vi "ActionVIOnCompile.vi"(8 "error in (no error)":errorcluster, 11 "Device Item Ref in":T1 format="%.0x") -> (0 "error out":errorcluster)   [LabVIEW 2019, in "NI-SWITCH System Explorer.lvlib"]
uses:
  NI-SWITCH System Explorer.lvlib
  <vilib>/NI VeriStand/Custom Device API/Custom Device Item Ref.ctl
  Shared/Compiled.Settings.ctl
  Shared/Communication Configuration.ctl
  Shared/Driver Configuration.ctl
  Shared/FIFO Indices.ctl
  Shared/Constants.vi
  <vilib>/NI VeriStand/Custom Device API/Set Item Property (Variant).vi
  <vilib>/NI VeriStand/Custom Device API/Custom Device API.lvlib
  Shared/NI-SWITCH Shared.lvlib
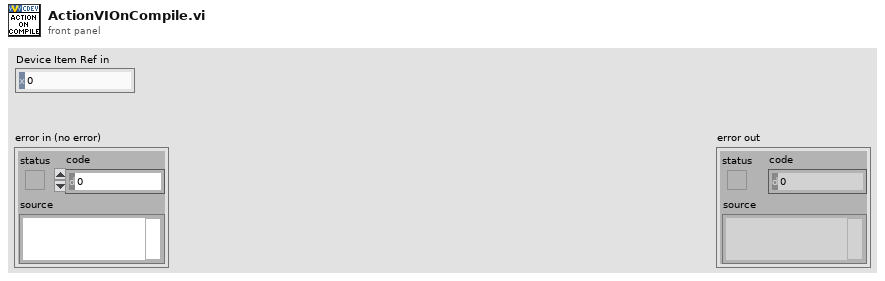
[diagram p1: front panel]
types:
  T1 = typedef "Custom Device API.lvlib/Custom Device Item Ref.ctl" = u64
  T2 = typedef "NI-SWITCH Shared.lvlib/Compiled.Settings.ctl" = cluster{"Custom Device Name":string, "Communication Configuration":T3, "Driver Configuration":T4, "FIFO Indices":T5}
  T3 = typedef "NI-SWITCH Shared.lvlib/Communication Configuration.ctl" = cluster{"Consumer Queue Name":string}
  T4 = typedef "NI-SWITCH Shared.lvlib/Driver Configuration.ctl" = cluster{"Topology":string, "Resource":string, "Source Channels":string[], "Configuration Channels":string[]}
  T5 = typedef "NI-SWITCH Shared.lvlib/FIFO Indices.ctl" = cluster{"Status Channel":i32, "Heartbeat Channel":i32}
  T6 = typedef "Custom Device API.lvlib/Custom Device Item Info.ctl" = cluster{"Name":string, "Is Channel":bool, "GUID":string, "Is Waveform":bool}
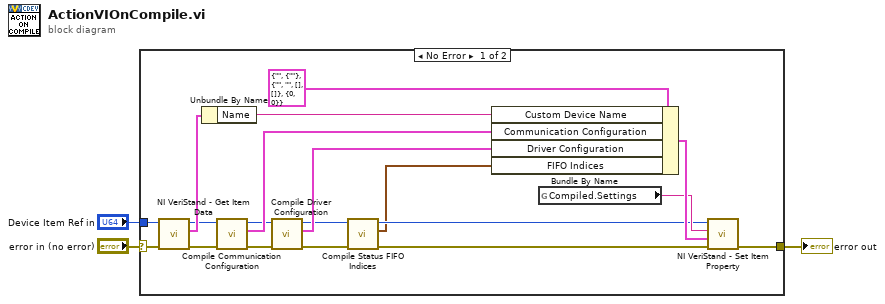
[diagram p0: block diagram]
diagram:
  n1 = case shown="No Error" "error in (no error)" {
    selector: "error in (no error)" -> [w21 w23]
    tunnel: [w22 w23] -> w2
    tunnel: "Device Item Ref in" -> [w20 _]
    frame No Error {
      n2 = call <vilib>:"NI VeriStand - Get Item Data.vi"("error in (no error)"=w21, "Item Ref in"=w20) -> ("error out"=w13:errorcluster, "Item Info"=w19:T6, "Item Ref out"=w14:T1)  [unwired: 6 in, 1 out]
      n3 = Unbundle By Name(w19) -> ("Name"=w18:string)
      n4 = call "Compile Communication Configuration.vi"("error in (no error)"=w13, "Device Ref in"=w14) -> ("error out"=w12:errorcluster, "Communication Configuration"=w11:T3, "Device Ref out"=w10:T1)  [unwired: 7 in]
      n5 = call "Compile Driver Configuration.vi"("error in (no error)"=w12, "Device Ref in"=w10) -> ("error out"=w8:errorcluster, "Driver Configuration"=w16:T4, "Device Ref out"=w7:T1)  [unwired: 7 in]
      n6 = call "Compile Status FIFO Indices.vi"("error in (no error)"=w8, "Device Item Ref in"=w7) -> ("error out"=w5:errorcluster, "FIFO Indices"=w4:T5, "Device Item Ref out"=w6:T1)  [unwired: 7 in]
      n7 = Bundle By Name(cluster=T2 {"Custom Device Name"="", "Communication Configuration"={"Consumer Queue Name"=""}, "Driver Configuration"={"Topology"="", "Resource"="", "Source Channels"=[], "Configuration Channels"=[]}, "FIFO Indices"={"Status Channel"=0, "Heartbeat Channel"=0}} ("Compiled.Settings"), "Custom Device Name"=w18, "Communication Configuration"=w11, "Driver Configuration"=w16, "FIFO Indices"=w4) -> (w15:T2)
      n8 = global read "Constants.vi" "Compiled.Settings"() -> (w9:string)
      n9 = call-poly <vilib>:"NI VeriStand - Set Item Property.vi"("error in (no error)"=w5, "Value"=w15, "Property Name"=w9, "Item Ref in"=w6) -> ("error out"=w22:errorcluster)  [unwired: 5 in, 2 out]
    }
    frame Error {
    }
  }
  "error out" <- w2
